vi "GEN_State Notifier.vi"(6 "Wait Time":u32, 7 "Action Select":T1(ring)=enum."Send Notification", 8 "error in (no error)":errorcluster caption="错误输入（无错误）", 10 "Notification":string, 11 "Notifier Name":string) -> (0 "error out":errorcluster caption="错误输出", 3 "Notification out":string)   [LabVIEW 2016]
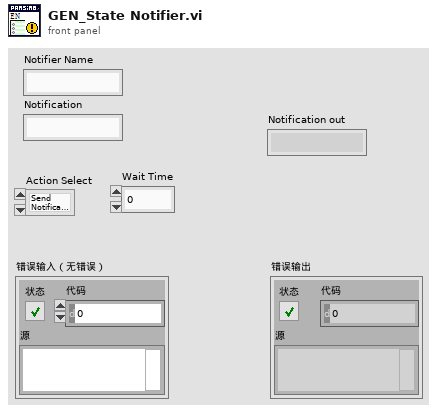
[diagram p1: front panel]
types:
  T1 = enum16{"Obtain Notifier", "Send Notification", "Wait Notification", "Release Notifier"}
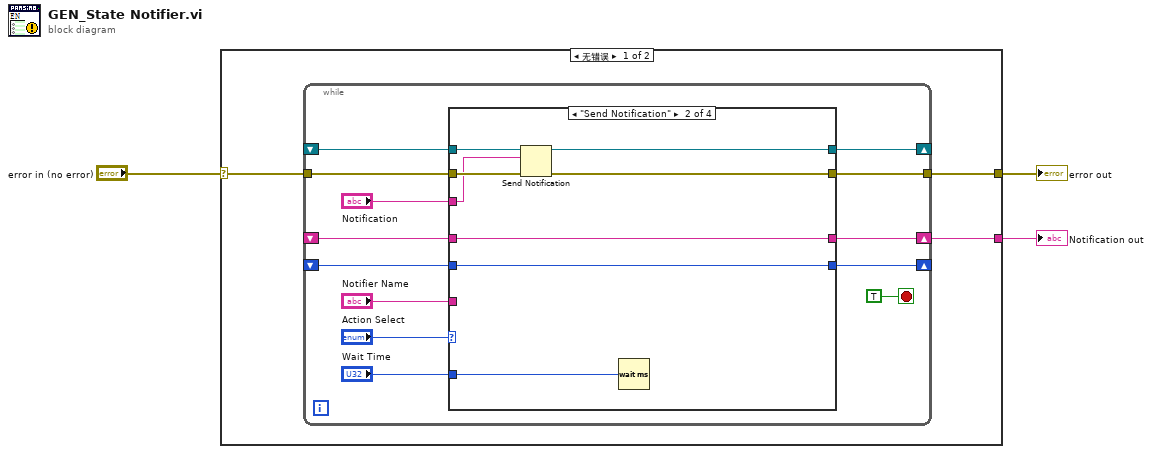
[diagram p0: block diagram]
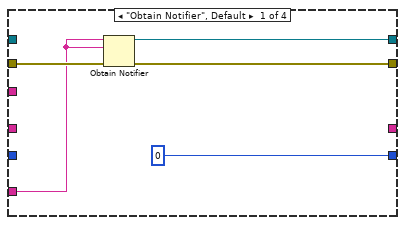
[diagram p2: hidden frame]
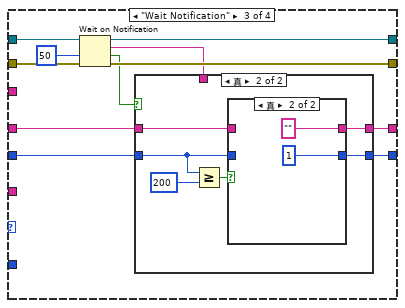
[diagram p3: hidden frame]
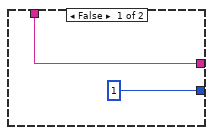
[diagram p4: hidden frame]
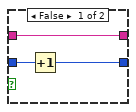
[diagram p5: hidden frame]
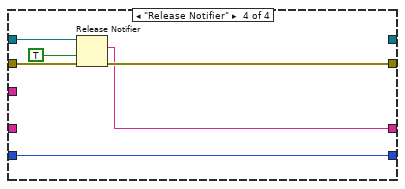
[diagram p6: hidden frame]
diagram:
  n1 = case shown="无错误" "error in (no error)" {
    selector: "error in (no error)" -> [w4 w63]
    tunnel: [w6 w63] -> w3
    tunnel: [w5 _] -> w2
    frame No Error {
      n2 = while {
        tunnel: w4 -> [w17]
        tunnel: [w16] -> w6
        shift-right: [w15] -> _
        shift-left: _ -> [w14]
        shift-right: [w12] -> w5
        shift-left: _ -> [w10]
        shift-right: [w8] -> _
        shift-left: _ -> [w9]
        stop <- TRUE stop-if-true
        n3 = case shown="\"Send Notification\"" "Action Select" {
          tunnel: "Notifier Name" -> [w22 _ _ _]
          tunnel: w17 -> [w24 w32 w43 w62]
          tunnel: [w23 w29 w40 w60] -> w16
          tunnel: [w21 w28 w39 _] -> w15
          tunnel: w14 -> [_ w31 w42 w61]
          tunnel: "Notification" -> [_ w30 _ _]
          tunnel: [_ w27 w34 w58] -> w12
          tunnel: w10 -> [_ w27 w36 _]
          tunnel: w9 -> [_ w26 w37 w57]
          tunnel: [0 w26 w35 w57] -> w8
          tunnel: "Wait Time" -> [_ w25 _ _]
          frame "Obtain Notifier", Default {
            n4 = Obtain Notifier ("获取通知器引用")(name (unnamed)=w22, notification data type=w22, error in (no error)=w24) -> (notifier out=w21:refnum<notifier>, error out=w23:errorcluster)  [unwired: 1 in, 1 out]
          }
          frame "Send Notification" {
            n5 = Send Notification(notification=w30, notifier=w31, error in (no error)=w32) -> (notifier out=w28:refnum<notifier>, error out=w29:errorcluster)
            n6 = Wait (ms)(milliseconds to wait=w25) -> ()  [unwired: 1 out]
          }
          frame "Wait Notification" {
            n7 = Wait on Notification(notifier=w42, timeout in ms (-1)=50 ("超时毫秒(-1)"), error in (no error)=w43) -> (notifier out=w39:refnum<notifier>, notification=w33:string, timed out?=w38:bool, error out=w40:errorcluster)  [unwired: 1 in]
            n8 = case shown="真" w38 {
              tunnel: w37 -> [_ w50]
              tunnel: w36 -> [_ w49]
              tunnel: [1 w48] -> w35
              tunnel: [w44 w47] -> w34
              tunnel: w33 -> [w44 _]
              frame False {
              }
              frame True {
                n9 = Greater Or Equal?(x=w50, y=200) -> (x >= y?=w51:bool)
                n10 = case shown="真" w51 {
                  tunnel: w50 -> [w54 _]
                  tunnel: w49 -> [w53 _]
                  tunnel: [w52 1] -> w48
                  tunnel: [w53 "" ("Notifier Name")] -> w47
                  frame False {
                    n11 = Increment(x=w54) -> (x+1=w52:i32)
                  }
                  frame True {
                  }
                }
              }
            }
          }
          frame "Release Notifier" {
            n12 = Release Notifier(notifier=w61, force destroy? (F)=TRUE ("强制销毁？(F)"), error in (no error)=w62) -> (last notification=w58:string, error out=w60:errorcluster)  [unwired: 1 out]
          }
        }
      }
    }
    frame Error {
    }
  }
  "error out" <- w3
  "Notification out" <- w2
